vi "AlliGator Source Image ROI Storage [MULT] v3.vi"(7 "Curent ROI Colors":u32[](array[colorbox]), 8 "Error In":errorcluster, 9 "Current ROI Descriptors":T2[](array[typedef]) {"Contours"."Type" items=["No Selection", "Point", "Line", "Rectangle", "Oval", "Polygon", "Freehand Region", "Annulus", "Unused2", "Unused3", "Broken Line", "Freehand Line", "Rotated Rectangle"]}, 10 "Default Names (\"ROI\")":string[](array[string]), 11 "Action":T1=enum."Update Current ROI Descriptor") -> (0 "Error Out":errorcluster, 1 "Current ROI Descriptors":T2[](array[typedef]) {"Contours"."Type" items=["No Selection", "Point", "Line", "Rectangle", "Oval", "Polygon", "Freehand Region", "Annulus", "Unused2", "Unused3", "Broken Line", "Freehand Line", "Rotated Rectangle"]}, 2 "Current ROI Names":string[](array[string]), 3 "Current Source Image ROI":i32, 4 "Old ROI Name":string, 5 "Curent ROI Colors":u32[](array[colorbox]))   [LabVIEW 2021, in "AlliGator ROIs.lvlib"]
doc: "Handles multiple Source Image ROIs storage."
uses:
  AlliGator ROIs.lvlib
  Image/Named ROI Description.ctl
  Image/Image.lvlib
  AlliGator Globals, Variables & Constants.lvlib
  AlliGator Variables List.ctl
  Variant/Variant to Data/Variant to Data.lvlib
  <userlib>/_OpenG.lib/array/array.llb/openg_array.lvlib
  Strings/Strings.lvlib
  <userlib>/_OpenG.lib/array/array.llb/Sort 1D Array (I32)__ogtk.vi
  Variant/Variant to Data/Variant to I32.vi
  AlliGator ROI Manager Actions.ctl
  Utilities/Utilities.lvlib
panel:
  # "see the AlliGator License on the block diagram (Ctrl+E or Window:Show Block Diagram)"
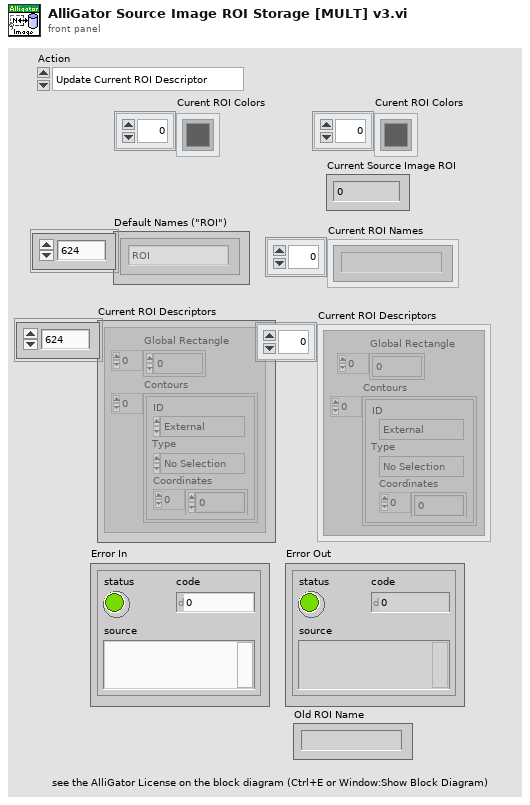
[diagram p1: front panel]
types:
  T1 = typedef "AlliGator ROIs.lvlib/AlliGator ROI Manager Actions.ctl" = enum16{"Undefined", "Delete Current ROI", "Delete All Unselected ROIs", "Delete Multiple ROIs", "Delete All ROIs", "Swap ROIs", "Insert ROI", "Update Current ROI Descriptor", "Rename Current ROI", "Store New ROI", "Store Multiple ROIs", "Select Next ROI", "Select Previous ROI", "Find Selected ROI", "Show All ROIs", "Update ROI Manager Window", "Merge All ROIs", "Unmerge ROI", "Set Selected ROI by ID"}
  T2 = typedef "ROI Descriptor" = cluster{"Global Rectangle":i32[], "Contours":cluster{"ID":enum32{"External", "Internal"}, "Type":u32, "Coordinates":i32[]}[]}
  T3 = typedef "AlliGator Globals, Variables & Constants.lvlib/AlliGator Variables List.ctl" = enum16{"---- GUI ----", "GUI:Initialization Status", "GUI:State Indicators Refnum", "GUI:Original AlliGator Menu Items", "GUI:Current Action Loop State", "GUI:Script in progress", "GUI:Playback", "GUI:Loop Playback", "GUI:Search ROI Used", "GUI:Search ROI", "Decay Graph Max Legend Size", "Intensity Graph Max Legend Size", "Decay Statistics Graph Max Legend Size", "Phasor Graph Max Legend Size", "Phasor Ratio Graph Max Legend Size", "Lifetime Graph Max Legend Size", "---- Files ----", "Files:Export Dataset Frames as Individual Files", "Files:Show Batch Export Help Balloons", "Files:Frames in Dataset", "Files:ptu File Frame Start Indices", "Files:Current Frame in Dataset", "Files:Current Frame Timestamp", "Files:Dataset Loaded", "Files:Dataset Metadata", "Files:Dataset Channel", "Files:Dataset Data Description", "Files:Background Dataset Metadata", "Files:Background Dataset Channel", "Files:Background Dataset Data Description", "Files:Background File Subtraction", "Files:Background File Path", "Files:Background File Pile-up Correction", "Files:Background File Pixel Well Capacity", "Files:Background File Scaling Factor", "Files:Current Dataset Load Settings", "Files:Dataset Path", "------ Python Plugins ------", "Python Plugins:Information", "Python Plugins:Python Session", "Python Plugins:Valid Python Session?", "---- Source Image ----", "Source Image:ROIs", "Source Image:Current ROI", "Source Image ROI Event Refnum", "X_Source Image Display Range", "X_Source Image Palette Information", "Source Image:Palette List", "Source Image:Scale", "Source Image:ROI Overlay Color", "Source Image:ICCD-specific Information", "---- Image Profile Window ----", "Image Profile:Overlay ROI in Source Image", "Image Profile Window Event Refnum", "Image Profile:IntensityType", "Image Profile:Intensity Average Type", "Image Profile:Intensity-weighted SDV", "Image Profile:Box Profile Type", "Image Profile Window Open", "Image Profile:Plotted Fit Parameter", "X_Type of Displayed Image", "X_Time Gate Slider", "Source Image:Overlay to Erase", "Is Displayed Image Accumulated", "White Light Image Modified", "Mask Image Modified", "Macrotime Gate Separation", "------ Phasor Graph -------", "Phasor Graph:Show Line", "---- Phasor Plot ---", "Phasor Plot Parameters Changed", "FLI Dataset Modified since last Phasor Plot Calculation", "Phasor Harmonics Data", "Selected Phasor Harmonics", "Phasor Harmonic Manager Event Refnum", "Phasor Plot ROIs", "Current Phasor Plot ROI", "Phasor Plot ROI Event Refnum", "Phasor Plot Image Reference Points", "Phasor Plot Computed", "Phasor Plot Palette Information", "Phasor Plot Palette List", "Phasor Ratio Palette Information", "Phasor Ratio Palette List", "Phasor Image Scale", "Phasor Plot Image Overlay to Erase", "Phasor Plot Image Elements to Update", "Current Phasor Plot Calculation Parameters", "Current Phasor Calibration Options", "Reset Cumulated Phasor Plot", "Phasor Ratio Reference 1", "Phasor Ratio Lifetime Reference 1", "Phasor Ratio Reference 1 Frequency", "Phasor Ratio Reference 2", "Phasor Ratio Lifetime Reference 2", "Phasor Ratio Reference 2 Frequency", "---- Decay Analysis ----", "Number of Selected Decays to Fit", "LS Fit Results", "LAR Fit Results", "BS Fit Results", "Last Decay Max - Min", "Best Fit Parameters", "Best Fit Parameter Names", "Actual Size X", "Actual Size Y", "Binning X", "Binning Y", "Actual # Gates", "Dataset Number", "Gates to...", "Gates Skipped", "Gates to keep", "Gate Step", "Gate Separation", "Reversed Gates", "Pile-up Correction", "Pixel Well Capacity", "Background Subtracted", "Background Subtraction Method", "Background Definition Range", "Background File (deprecated)", "Number of Dataset Accumulated", "Array of Accumulated Dataset Paths", "Do Averaged Datasets", "Destination File Path", "Process Plot Target", "Use 1/D as Phasor Frequency", "---- Decay Fit Parameter Map -----", "Decay Fit Parameter Map Palette Information", "Decay Fit Parameter Map Palette List", "Local Decay Graph Window Event Refnum", "------- Local Decay Window ---------", "Use normalized IRF for convolution", "----- Miscellaneous ----", "Skippable Dialog Windows Status"}
  T4 = typedef "Image.lvlib/Named ROI Description.ctl" = cluster{"ROI Descriptor":T2, "ROI Name":string, "Overlay Color":u32}
  T5 = typedef "AlliGator ROIs.lvlib/AlliGator Image ROI Event refnum.ctl" = refnum<user-event>
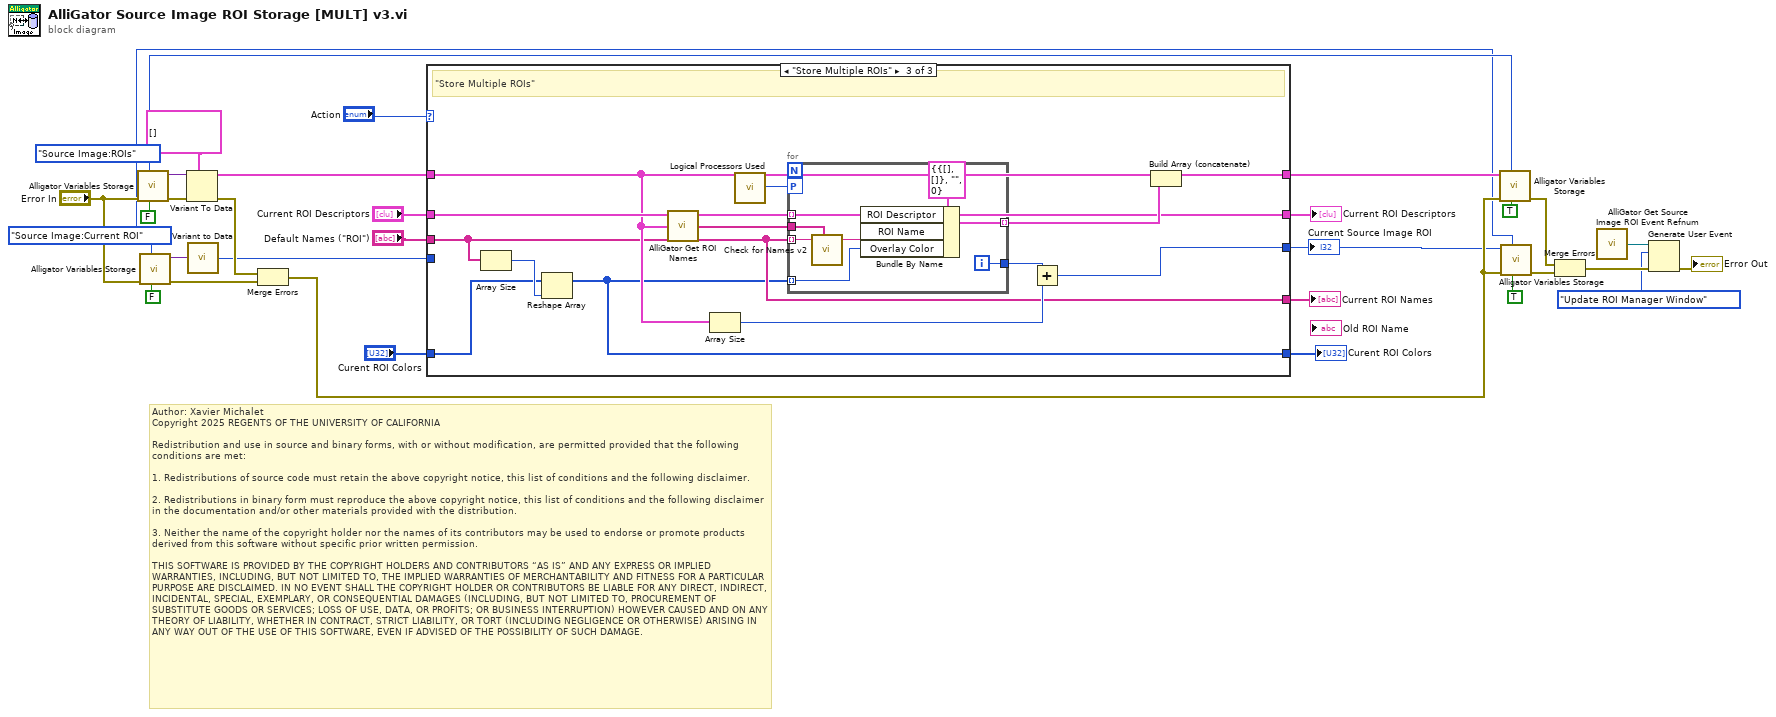
[diagram p0: block diagram]
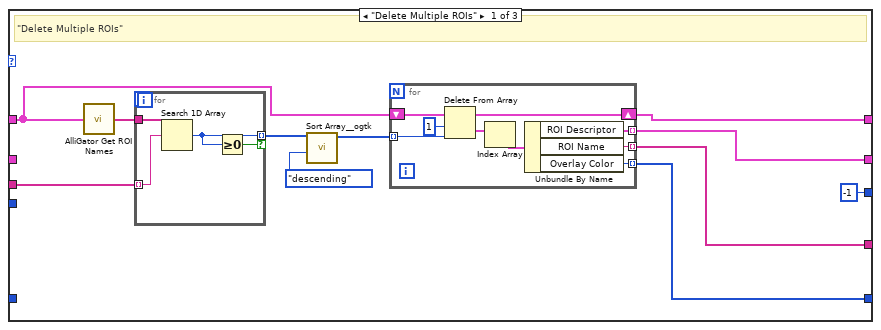
[diagram p2: hidden frame]
diagram:
  w1 = AlliGator_Variables_List."Source Image:Current ROI" ("Alligator Variable")
  w2 = AlliGator_Variables_List."Source Image:ROIs" ("Alligator Variable")
  # "Author: Xavier Michalet\nCopyright 2025 REGENTS OF THE UNIVERSITY OF CALIFORNIA\n\nRedistribution and use in source and binary forms, with or without modification, are permitted provided that the following conditions are met:\n\n1. Redistributions of source code must retain the above copyright notice, this list of conditions and the following disclaimer.\n\n2. Redistributions in binary form must reproduce the above copyright notice, this list of conditions and the following disclaimer in the documentation and/or other materials provided with the distribution.\n\n3. Neither the name of the copyright holder nor the names of its contributors may be used to endorse or promote products derived from this software without specific prior written permission.\n\nTHIS SOFTWARE IS PROVIDED BY THE COPYRIGHT HOLDERS AND CONTRIBUTORS “AS IS” AND ANY EXPRESS OR IMPLIED WARRANTIES, INCLUDING, BUT NOT LIMITED TO, THE IMPLIED WARRANTIES OF MERCHANTABILITY AND FITNESS FOR A PARTICULAR PURPOSE ARE DISCLAIMED. IN NO EVENT SHALL THE COPYRIGHT HOLDER OR CONTRIBUTORS BE LIABLE FOR ANY DIRECT, INDIRECT, INCIDENTAL, SPECIAL, EXEMPLARY, OR CONSEQUENTIAL DAMAGES (INCLUDING, BUT NOT LIMITED TO, PROCUREMENT OF SUBSTITUTE GOODS OR SERVICES; LOSS OF USE, DATA, OR PROFITS; OR BUSINESS INTERRUPTION) HOWEVER CAUSED AND ON ANY THEORY OF LIABILITY, WHETHER IN CONTRACT, STRICT LIABILITY, OR TORT (INCLUDING NEGLIGENCE OR OTHERWISE) ARISING IN ANY WAY OUT OF THE USE OF THIS SOFTWARE, EVEN IF ADVISED OF THE POSSIBILITY OF SUCH DAMAGE."
  n1 = call "Alligator Variables Storage.vi"("Get(F)/Set"=FALSE, "AlliGator Variable"=w2, "Error In"="Error In") -> ("Error Out"=w30:errorcluster, "Data out"=w31:variant)  [unwired: 6 in, 1 out]
  n2 = call "Alligator Variables Storage.vi"("Get(F)/Set"=FALSE, "AlliGator Variable"=w1, "Error In"="Error In") -> ("Error Out"=w22:errorcluster, "Data out"=w26:variant)  [unwired: 6 in, 1 out]
  n3 = Variant To Data(error in=w30, type=T4[] [] ("Stored ROIs in"), Variant=w31) -> (data=w15:T4[], error out=w21:errorcluster)
  n4 = call-poly "Variant to Data.vi"("Variant"=w26) -> ("Value"=w14:i32)  [unwired: 8 in]
  n5 = Merge Errors(w21, w22) -> (w16:errorcluster)
  n6 = case shown="\"Store Multiple ROIs\"" "Action" {
    tunnel: w15 -> [w38 w59 w66]
    tunnel: w14 -> [_ w57 _]
    tunnel: [w37 w59 w72] -> w11
    tunnel: [-1 w57 w67] -> w10
    tunnel: "Current ROI Descriptors" -> [_ w58 w70]
    tunnel: [w35 w58 w70] -> w9
    tunnel: "Default Names (\"ROI\")" -> [w41 _ w64]
    tunnel: [w33 _ w64] -> w8
    tunnel: [w32 w56 w61] -> w7
    tunnel: "Curent ROI Colors" -> [_ w56 w62]
    frame "Delete Multiple ROIs" {
      # "\"Delete Multiple ROIs\""
      n7 = call "AlliGator Get ROI Names.vi"("Stored ROIs in"=w38) -> ("ROI Name"=w42:string[])  [unwired: 8 in]
      n8 = for {
        tunnel: w42 -> [w55]
        tunnel: w41 -> [w53] mode=indexing
        tunnel: [w54] -> w36 mode=indexing if=w52
        n9 = Search 1D Array(1D array=w55, element=w53) -> (index of element=w54:i32)  [unwired: 1 in]
        n10 = Greater Or Equal To 0?(x=w54) -> (x >= 0?=w52:bool)
      }
      n11 = call-poly <userlib>:"Sort Array__ogtk.vi"("Order"=enum16{"ascending", "descending"}."descending", "Array in"=w36) -> ("Sorted Array out"=w39:i32[])  [unwired: 8 in, 1 out]
      n12 = for {
        tunnel: w39 -> [w51] mode=indexing
        shift-right: [w48] -> w37
        shift-left: w38 -> [w49]
        tunnel: [w45] -> w35 mode=indexing
        tunnel: [w44] -> w33 mode=indexing
        tunnel: [w43] -> w32 mode=indexing
        n13 = Delete From Array(array=w49, length=1, index=w51) -> (deleted portion=w47:T4[], array with subset deleted=w48:T4[])
        n14 = Index Array(array=w47) -> (element=w46:T4)  [unwired: 1 in]
        n15 = Unbundle By Name(w46) -> ("ROI Descriptor"=w45:T2, "ROI Name"=w44:string, "Overlay Color"=w43:u32)
      }
    }
    frame Default {
    }
    frame "Store Multiple ROIs" {
      # "\"Store Multiple ROIs\""
      n16 = Array Size(array=w64) -> (size(s)=w63:i32)
      n17 = Reshape Array(w62, w63) -> (w61:u32[])
      n18 = call "AlliGator Get ROI Names.vi"("Stored ROIs in"=w66) -> ("ROI Name"=w65:string[])  [unwired: 8 in]
      n19 = Array Size(array=w66) -> (size(s)=w68:i32)
      n20 = call "Logical Processors Used.vi"() -> ("# Logical Processor Used"=w60:i32)  [unwired: 6 in]
      n21 = for {
        tunnel: w70 -> [w78] mode=indexing
        tunnel: [w79] -> w71 mode=indexing
        tunnel: w64 -> [w75] mode=indexing
        tunnel: [w77] -> w69
        tunnel: w65 -> [w76]
        tunnel: w61 -> [w73] mode=indexing
        workers-P: w60 -> [_]
        i -> [w77]
        n22 = call "Check for Names v2.vi"("New Name"=w75, "Name List"=w76) -> ("New Name"=w74:string)  [unwired: 4 in, 3 out]
        n23 = Bundle By Name(cluster=T4 {"ROI Descriptor"={"Global Rectangle"=[], "Contours"=[]}, "ROI Name"="", "Overlay Color"=0} ("Named ROI Description"), "ROI Descriptor"=w78, "ROI Name"=w74, "Overlay Color"=w73) -> (w79:T4)
      }
      n24 = Add(x=w69, y=w68) -> (x+y=w67:i32)
      n25 = Build Array (concatenate)(w66, w71) -> (w72:T4[])
    }
  }
  "Current ROI Descriptors" <- w9
  "Current Source Image ROI" <- w10
  "Current ROI Names" <- w8
  "Curent ROI Colors" <- w7
  n26 = call "Alligator Variables Storage.vi"("Get(F)/Set"=TRUE, "AlliGator Variable"=w2, "Error In"=w16, "Data in"=w11) -> ("Error Out"=w19:errorcluster)  [unwired: 5 in, 2 out]
  n27 = call "Alligator Variables Storage.vi"("Get(F)/Set"=TRUE, "AlliGator Variable"=w1, "Error In"=w16, "Data in"=w10) -> ("Error Out"=w20:errorcluster)  [unwired: 5 in, 2 out]
  n28 = Merge Errors(w19, w20) -> (w18:errorcluster)
  n29 = call "AlliGator Get Source Image ROI Event Refnum.vi"() -> ("Source Image ROI Event Refnum"=w4:T5)
  n30 = Generate User Event(user event=w4, event data cluster=AlliGator_ROI_Manager_Actions."Update ROI Manager Window" ("event data"), error in=w18) -> (error out=→"Error Out":errorcluster)  [unwired: 1 in, 1 out]
